vi "Start_Engine.vi"(0 "Host_Reference":refnum<class "HGF_Reference.lvclass">, 2 "timeout in ms (-1)":i32, 3 "HGF_Agent":refnum<class "MoAgSy_AgentBase.lvclass">, 5 "error in (no error)":errorcluster) -> (14 "dup Host_Reference":refnum<class "HGF_Reference.lvclass">, 16 "dup timeout in ms (-1)":i32, 19 "error out":errorcluster)   [LabVIEW 2009, in "MoAgSy.lvlib" / "MoAgSy_Host.lvclass"]
doc: "<B>public</B> VI runs Agent at referenced Host.\nFor that, a new Engine (task) is created and dispatched at Hosts threadpool.\n<B>Error Handling not yet implemented</B>\n\nF.Berck@gsi.de\nGSI Darmstadt 2009"
uses:
  MoAgSy_Host.lvclass
  HGF_BaseClasses/HGF_Reference/HGF_Reference.lvclass
  MoAgSy_AgentBase/MoAgSy_AgentBase.lvclass
  MoAgSy_Factory/MoAgSy_Factory.lvclass
  HGF_BaseClasses/HGF_ThreadTask/HGF_ThreadTask.lvclass
  HGF_BaseClasses/HGF_Factory/HGF_Factory.lvclass
  MoAgSy_Engine/MoAgSy_Engine.lvclass
  HGF_BaseClasses/HGF_ThreadPool/HGF_ThreadPool.lvclass
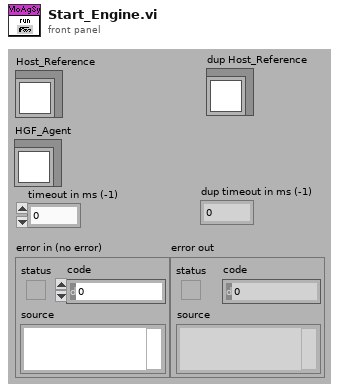
[diagram p1: front panel]
types:
  T1 = cluster{"Host Variable":refnum<k21>, "Agent_Event (Monitor Event)":refnum<class "HGF_Event.lvclass">, "Host_Event (Monitor Event)":refnum<class "HGF_Event.lvclass">, "DSCException":refnum<class "HGF_TriggeredEvent.lvclass">, "MoAgSy_DSCThreadPool":refnum<class "HGF_Reference.lvclass">, "ManagerEvent":refnum<class "HGF_Event.lvclass">, "DSCDestination":refnum<class "HGF_TriggeredEvent.lvclass">}
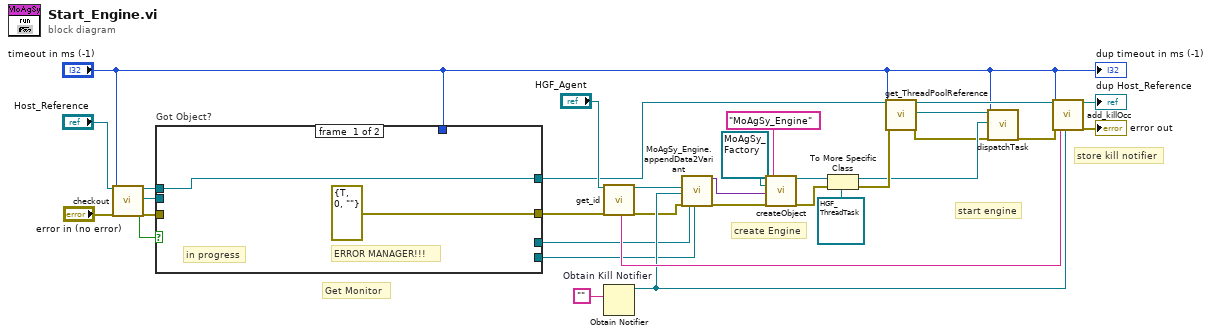
[diagram p0: block diagram]
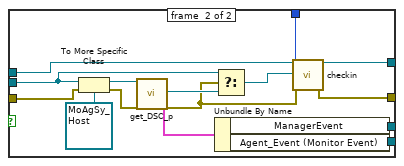
[diagram p2: hidden frame]
diagram:
  # "store kill notifier"
  # "start engine"
  # "create Engine"
  # "Get Monitor"
  n1 = call "checkout.vi"("HGF_Reference"="Host_Reference", "timeout in ms (-1)"="timeout in ms (-1)", "error in (no error)"="error in (no error)") -> ("dup HGF_Reference"=w12:refnum<class "HGF_Reference.lvclass">, "Object"=w9:refnum<class>, "got object?"=w8:bool, "error out"=w7:errorcluster)  [unwired: 13 out]
  n2 = case "Got Object?" shown="True" w8 {
    tunnel: w9 -> [_ w43]
    tunnel: w12 -> [w34 w48]
    tunnel: [w34 w47] -> w10
    tunnel: "timeout in ms (-1)" -> [_ w46]
    tunnel: [errorcluster {"status"=TRUE, "code"=0, "source"=""} ("error out") w45] -> w5
    tunnel: w7 -> [_ w44]
    tunnel: [_ w37] -> w4
    tunnel: [_ w35] -> w3
    frame #0 {
      # "in progress"
      # "ERROR MANAGER!!!"
    }
    frame #1 {
      n3 = To More Specific Class(target class=refnum<class "MoAgSy_Host.lvclass"> refnum ("MoAgSy.lvlib:MoAgSy_Host.lvclass"), reference=w43, error in=w44) -> (specific class reference=w41:refnum<class "MoAgSy_Host.lvclass">, error out=w36:errorcluster)
      n4 = call "get_DSC_p.vi"("MoAgSy_Host"=w41, "error in (no error)"=w36) -> ("dup MoAgSy_Host"=w40:refnum<class "MoAgSy_Host.lvclass">, "DSC"=w38:T1, "error out"=w39:errorcluster)  [unwired: 15 out]
      n5 = Unbundle By Name(w38) -> ("ManagerEvent"=w37:refnum<class "HGF_Event.lvclass">, "Agent_Event (Monitor Event)"=w35:refnum<class "HGF_Event.lvclass">)
      n6 = Select(t=w43, s=w39, f=w40) -> (s? t:f=w42:refnum<class>)
      n7 = call "checkin.vi"("HGF_Reference"=w48, "Object"=w42, "timeout /ms (-1)"=w46, "error in (no error)"=w39) -> ("dup HGF_Reference"=w47:refnum<class "HGF_Reference.lvclass">, "error out"=w45:errorcluster)  [unwired: 14 out]
    }
  }
  n8 = call "get_id.vi"("HGF_Agent in"="HGF_Agent", "error in (no error)"=w5) -> ("HGF_Agent out"=w20:refnum<class "MoAgSy_AgentBase.lvclass">, "ID"=w32:string, "error out"=w19:errorcluster)  [unwired: 15 out]
  n9 = Obtain Notifier "Obtain Kill Notifier"(notification data type="") -> (notifier out=w31:refnum<notifier>)  [unwired: 2 in, 3 out]
  n10 = call "MoAgSy_Engine.appendData2Variant.vi"("HGF_Agent"=w20, "kill notifier"=w31, "error in"=w19, "VarManagerEvent"=w4, "HGF_Event (Monitor Event)"=w3) -> ("dup init"=w28:variant, "error out"=w27:errorcluster)  [unwired: 2 in, 11 out]
  n11 = call "createObject.vi"("HGF_Factory"=refnum<class "MoAgSy_Factory.lvclass"> refnum ("MoAgSy.lvlib:MoAgSy_Factory.lvclass"), "initializationData"=w28, "error in (no error)"=w27, "className"="MoAgSy_Engine") -> ("HGF_Object"=w25:refnum<class "HGF_Factory.lvclass">, "error out"=w26:errorcluster)  [unwired: 1 in, 13 out]
  n12 = To More Specific Class(target class=refnum<class "HGF_ThreadTask.lvclass"> refnum ("HGF_BaseClasses.lvlib:HGF_ThreadTask.lvclass"), reference=w25, error in=w26) -> (specific class reference=w22:refnum<class "HGF_ThreadTask.lvclass">, error out=w24:errorcluster)
  n13 = call "get_ThreadPoolReference.vi"("Host_Reference"=w10, "timeout in ms (-1)"="timeout in ms (-1)", "error in (no error)"=w24) -> ("dup Host_Reference"=w18:refnum<class "HGF_Reference.lvclass">, "Threadpool Reference"=w2:refnum<class "HGF_Reference.lvclass">, "error out"=w1:errorcluster)  [unwired: 14 out]
  n14 = call "dispatchTask.vi"("HGF_ThreadPool_Reference"=w2, "HGF_ThreadTask"=w22, "timeout in ms (-1)"="timeout in ms (-1)", "error in (no error)"=w1) -> ("error out"=w16:errorcluster)  [unwired: 15 out]
  n15 = call "add_killOcc.vi"("Host_Reference"=w18, "timeout in ms (-1)"="timeout in ms (-1)", "error in (no error)"=w16, "ID"=w32, "killNotifier"=w31) -> ("dup Host_Reference"=→"dup Host_Reference":refnum<class "HGF_Reference.lvclass">, "error out"=→"error out":errorcluster)  [unwired: 2 in, 11 out]
  "dup timeout in ms (-1)" <- "timeout in ms (-1)"
